vi "Read Count.vi"(8 "error in (no error)":errorcluster, 11 "Count Request Message in":refnum<class "Count Request Message.lvclass">) -> (0 "error out":errorcluster, 2 "Count":u32, 3 "Count Request Message out":refnum<class "Count Request Message.lvclass">)   [LabVIEW 2017, in "Count Request Message.lvclass"]
uses:
  Count Request Message.lvclass
  Count Request Message.lvclass/Count Request Message.ctl
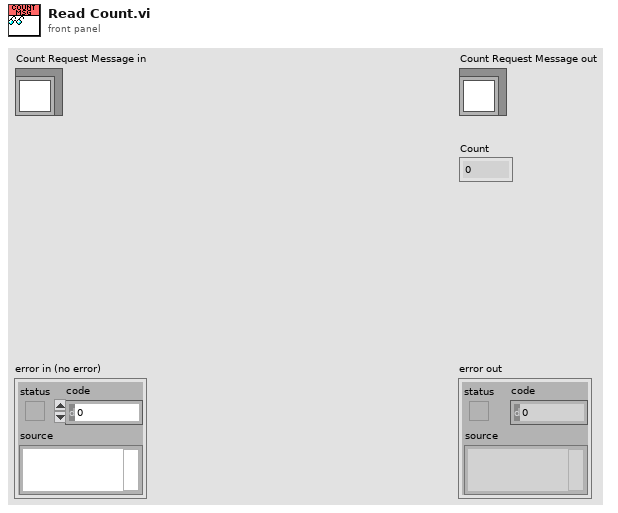
[diagram p1: front panel]
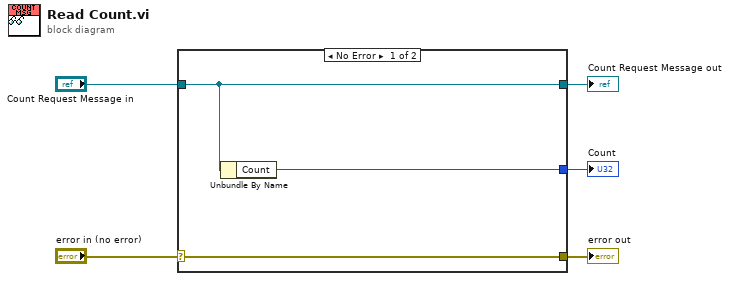
[diagram p0: block diagram]
diagram:
  n1 = case shown="No Error" "error in (no error)" {
    selector: "error in (no error)" -> [w8 w9]
    tunnel: [w8 w9] -> w4
    tunnel: [w7 w10] -> w2
    tunnel: "Count Request Message in" -> [w7 w10]
    tunnel: [w6 _] -> w1
    frame No Error {
      n2 = Unbundle By Name(w7) -> ("Count"=w6:u32)
    }
    frame Error {
    }
  }
  "error out" <- w4
  "Count Request Message out" <- w2
  "Count" <- w1
